vi "Configure IQ Adjustment External.vi"(0 "VISA resource name":refnum<visa-resource-name>, 1 "Differential Mode Q Offset (0 V)":dbl, 2 "Differential Mode I Offset (0 V)":dbl, 3 "Common Mode I/Q Offset (0 V)":dbl, 5 "External I Offset (0 V)":dbl, 7 "External Q Offset (0 V)":dbl, 9 "External Gain (0 dB)":dbl, 11 "error in (no error)":errorcluster, 12 "Attenuation Level (6 dB)":dbl=6.0, 13 "Quadrature Angle Adjustment (0 deg)":dbl) -> (4 "VISA resource name out":refnum<visa-resource-name>, 15 "error out":errorcluster)   [LabVIEW 2009, in "Agilent PSG MXG Series.lvlib"]
doc: "Configures external I/Q adjustments.\n\n<B>Notes:</B>\n(1) This VI is valid only in E8267C, E8267D, N5182A.\n\n(2) For E8267C, this VI is valid only when the instrument installs <B>Option 002</B> (Internal baseband generator) or <B>Option 602</B> (Digital bus baseband generator)."
uses:
  Agilent PSG MXG Series.lvlib
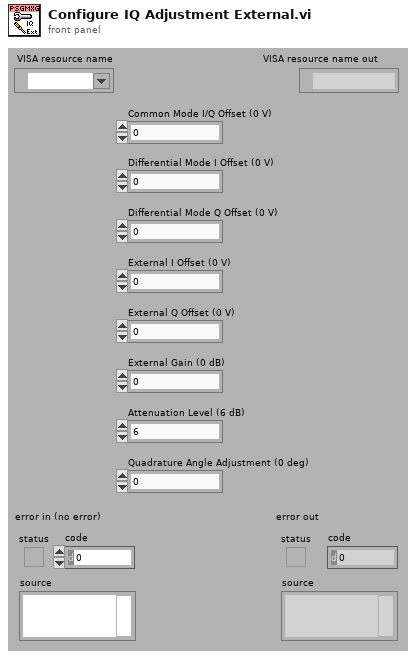
[diagram p1: front panel]
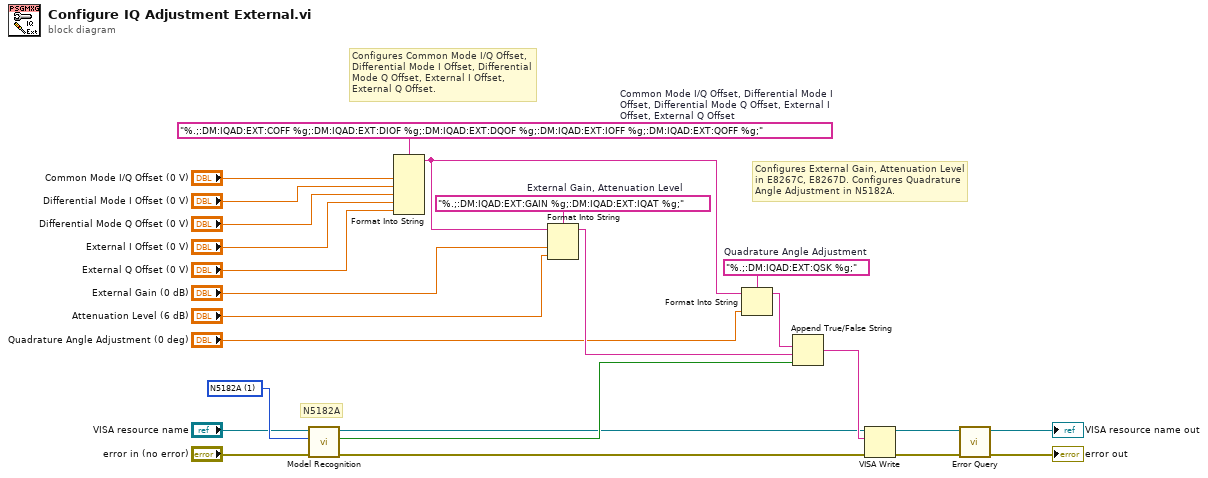
[diagram p0: block diagram]
diagram:
  w8 = u16 1 items=["N5181A"=0, "N5182A"=1, "E8241A"=5, "E8244A"=6, "E8251A"=7, "E8254A"=8, "E8247C"=10, "E8257C"=11, "E8267C"=12, "E8257D"=15, "E8267D"=16] ("Model Type (0: N5181A)")
  w14 = "%.;:DM:IQAD:EXT:QSK %g;"  # Quadrature Angle Adjustment
  w24 = "%.;:DM:IQAD:EXT:GAIN %g;:DM:IQAD:EXT:IQAT %g;"  # External Gain, Attenuation Level
  w25 = "%.;:DM:IQAD:EXT:COFF %g;:DM:IQAD:EXT:DIOF %g;:DM:IQAD:EXT:DQOF %g;:DM:IQAD:EXT:IOFF %g;:DM:IQAD:EXT:QOFF %g;"  # Common Mode I/Q Offset, Differential Mode I Offset, Differential Mode Q Offset, External I Offset, External Q Offset
  # "Configures External Gain, Attenuation Level\nin E8267C, E8267D. Configures Quadrature\nAngle Adjustment in N5182A."
  # "Configures Common Mode I/Q Offset,\nDifferential Mode I Offset, Differential\nMode Q Offset, External I Offset,\nExternal Q Offset."
  # "N5182A"
  n1 = call "Model Recognition.vi"("error in (no error)"="error in (no error)", "Model Type (0: N5181A)"=w8, "VISA resource name"="VISA resource name") -> ("error out"=w5:errorcluster, "Is Model Correct"=w7:bool, "VISA resource name out"=w6:refnum<visa-resource-name>)  [unwired: 6 out]
  n2 = Format Into String(format string=w25, "Common Mode I/Q Offset (0 V)", "Differential Mode I Offset (0 V)", "Differential Mode Q Offset (0 V)", "External I Offset (0 V)", "External Q Offset (0 V)") -> (resulting string=w15:string)  [unwired: 2 in, 1 out]
  n3 = Format Into String(format string=w24, initial string=w15, "External Gain (0 dB)", "Attenuation Level (6 dB)") -> (resulting string=w18:string)  [unwired: 1 in, 1 out]
  n4 = Format Into String(format string=w14, initial string=w15, "Quadrature Angle Adjustment (0 deg)") -> (resulting string=w13:string)  [unwired: 1 in, 1 out]
  n5 = Append True/False String(1:w7, 2:w18, 3:w13) -> (0:w11:string)  [unwired: 1 out]
  n6 = VISA Write(VISA resource name=w6, write buffer=w11, error in (no error)=w5) -> (VISA resource name out=w10:refnum<visa-resource-name>, error out=w9:errorcluster)  [unwired: 1 out]
  n7 = call "Error Query.vi"("error in (no error)"=w9, "VISA resource name"=w10) -> ("error out"=→"error out":errorcluster, "VISA resource name out"=→"VISA resource name out":refnum<visa-resource-name>)  [unwired: 8 out]
